vi "ReadFromDictionary.vi"(7 "Section":string[](array[string]), 8 "error in (no error)":errorcluster, 10 "Keys":string[](array[string]), 11 "ConfigManager.Text in":refnum<class "ConfigManager.Text.lvclass">) -> (0 "error out":errorcluster, 1 "Values":string[](array[string]), 2 "Keys out":string[](array[string]), 3 "ConfigManager.Text out":refnum<class "ConfigManager.Text.lvclass">, 4 "Found":bool[](array[boolean]), 5 "Section":string[](array[string]))   [LabVIEW 2013, in "CfgManager.Text.lvlib" / "ConfigManager.Text.lvclass"]
uses:
  ConfigManager.Text.lvclass
  ConfigManager.Text.lvclass/ConfigManager.Text.ctl
  <vilib>/LabVIEW Open Source Project/Unicity/Delimiter/Delimiter.lvclass
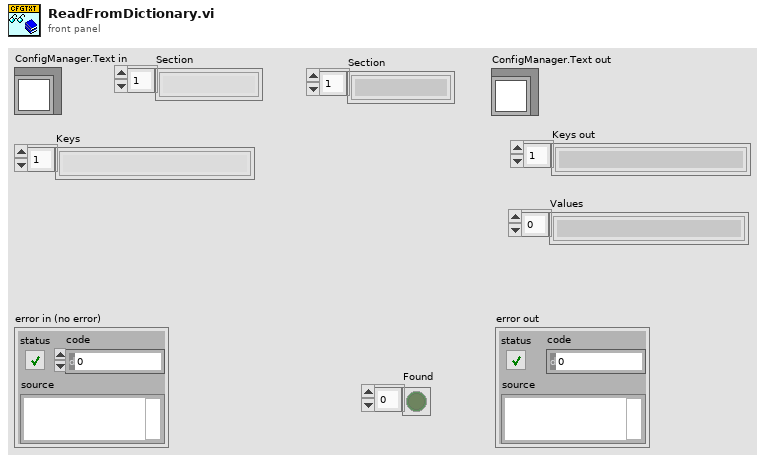
[diagram p1: front panel]
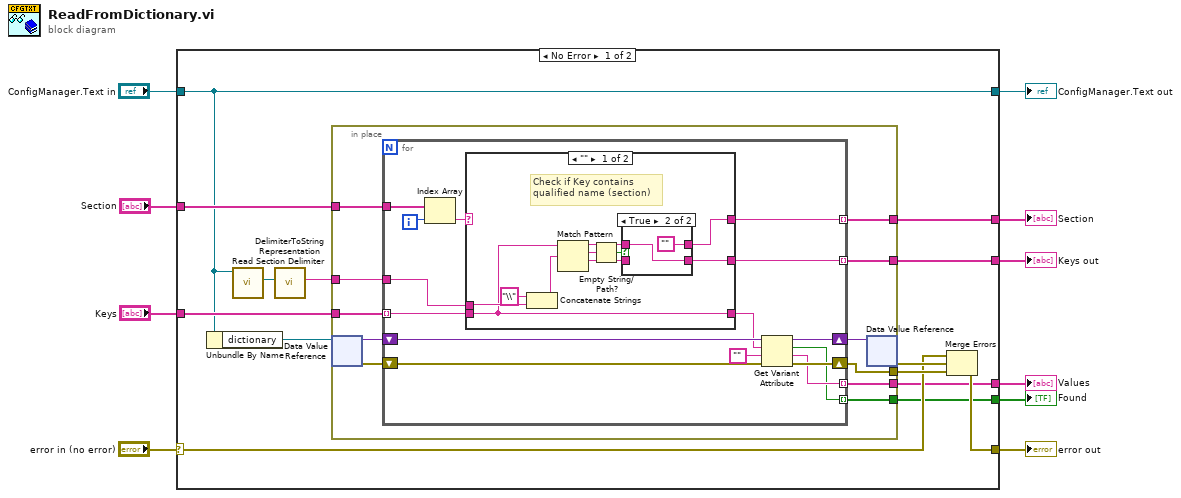
[diagram p0: block diagram]
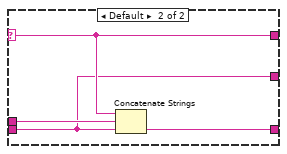
[diagram p3: hidden frame]
diagram:
  n1 = case shown="No Error" "error in (no error)" {
    selector: "error in (no error)" -> [w20 w71]
    tunnel: [w24 w71] -> w10
    tunnel: "Keys" -> [w15 w69]
    tunnel: "ConfigManager.Text in" -> [w12 w70]
    tunnel: [w12 w70] -> w7
    tunnel: [w19 _] -> w6
    tunnel: "Section" -> [w16 _]
    tunnel: [w18 _] -> w3
    tunnel: [w14 _] -> w2
    tunnel: [w13 w69] -> w1
    frame No Error {
      n2 = Unbundle By Name(w12) -> ("dictionary"=w21:refnum<data-value>)
      n3 = call "Read Section Delimiter.vi"("ConfigManager.Text in"=w12) -> ("Section Delimiter"=w11:refnum<class "Delimiter.lvclass">)  [unwired: 9 in, 1 out]
      n4 = call <vilib>:"DelimiterToStringRepresentation.vi"("Delimiter"=w11) -> ("String representation"=w17:string)  [unwired: 10 in]
      n5 = in-place {
        in-place-border: w15 -> [w30]
        in-place-border: [w32] -> w23
        in-place-border: [w31] -> w19
        in-place-border: [w29] -> w18
        in-place-border: w17 -> [w28]
        in-place-border: w16 -> [w27]
        in-place-border: [w26] -> w14
        in-place-border: [w25] -> w13
        n6 = in-place-dvr #1(w21) -> (w35:variant, w33:errorcluster)
        n7 = for {
          shift-right: [w49] -> w34
          shift-left: w35 -> [w50]
          tunnel: w30 -> [w43] mode=indexing
          shift-right: [w47] -> w32
          shift-left: w33 -> [w48]
          tunnel: [w45] -> w31 mode=indexing
          tunnel: [w44] -> w29 mode=indexing
          tunnel: w28 -> [w42]
          tunnel: w27 -> [w41]
          tunnel: [w38] -> w26 mode=indexing
          tunnel: [w37] -> w25 mode=indexing
          i -> [w40]
          n8 = Index Array(array=w41, index=w40) -> (element=w39:string)
          n9 = case shown="\"\"" w39 {
            selector: w39 -> [_ w66]
            tunnel: w43 -> [w51 w65]
            tunnel: [w51 w68] -> w36
            tunnel: w42 -> [w52 w67]
            tunnel: [w54 w66] -> w38
            tunnel: [w53 w65] -> w37
            frame "" {
              # "Check if Key contains\nqualified name (section)"
              n10 = Concatenate Strings("\\" ("string"), w52) -> (w60:string)
              n11 = Match Pattern(string=w51, regular expression=w60) -> (before substring=w56:string, match substring=w58:string, after substring=w55:string)  [unwired: 1 in, 1 out]
              n12 = Empty String/Path?(string/path=w58) -> (empty?=w57:bool)
              n13 = case shown="True" w57 {
                tunnel: [w61 w64] -> w53
                tunnel: w56 -> [w62 w64]
                tunnel: w55 -> [w61 _]
                tunnel: [w62 ""] -> w54
                frame False {
                }
                frame True {
                }
              }
            }
            frame Default {
              n14 = Concatenate Strings(w66, w67, w65) -> (w68:string)
            }
          }
          n15 = Get Variant Attribute(Variant=w50, name=w36, default value (empty Variant)="", error in=w48) -> (duplicate Variant=w49:variant, found=w44:bool, value=w45:string, error out=w47:errorcluster)
        }
        n16 = in-place-dvr #1(w34) -> (w22:errorcluster)  [unwired: 1 out]
      }
      n17 = Merge Errors(w20, w22, w23) -> (w24:errorcluster)
    }
    frame Error {
    }
  }
  "error out" <- w10
  "Values" <- w6
  "ConfigManager.Text out" <- w7
  "Keys out" <- w1
  "Found" <- w3
  "Section" <- w2
